vi "Get Parameter.vi"(8 "error in (no error)":errorcluster, 11 "request in":refnum<class "request.lvclass">) -> (0 "error out":errorcluster, 2 "parameter":variant, 3 "request out":refnum<class "request.lvclass">)   [LabVIEW 2015, in "request.lvclass"]
uses:
  request.lvclass
  request.lvclass/request.ctl
  <vilib>/addons/lv-msgpack/MsgPack Deserializer/MsgPackDeserializer.lvclass
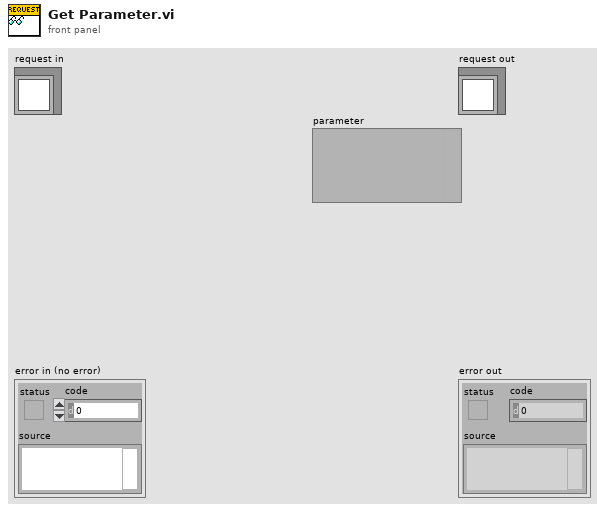
[diagram p1: front panel]
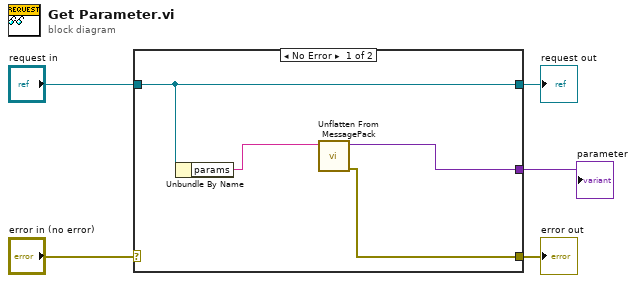
[diagram p0: block diagram]
diagram:
  n1 = case shown="No Error" "error in (no error)" {
    selector: "error in (no error)" -> [_ w10]
    tunnel: [w7 w10] -> w4
    tunnel: [w9 w11] -> w2
    tunnel: "request in" -> [w9 w11]
    tunnel: [w6 _] -> w1
    frame No Error {
      n2 = Unbundle By Name(w9) -> ("params"=w8:string)
      n3 = call <vilib>:"Unflatten From MessagePack.vi"("MsgPack Data"=w8) -> ("error IO"=w7:errorcluster, "Data"=w6:variant)  [unwired: 8 in, 1 out]
    }
    frame Error {
    }
  }
  "error out" <- w4
  "request out" <- w2
  "parameter" <- w1
